vi "MC Cycle Engine Request State ERD.vi"(0 "GEA2 Reference In":refnum<k24>, 1 "GEA Inputs":T2 {"Destination" format="%.0x"; "Source" format="%.0x"}, 2 "Standalone?":bool, 7 "Cycle #":u8, 9 "MC Cycle Engine State":T1, 11 "Error In":errorcluster) -> (4 "GEA2 Reference Out":refnum<k24>, 15 "Error Out":errorcluster)   [LabVIEW 2016, in "TL27.lvlib"]
doc: "This vi can be used to update the MC cycle engine state with the requested values."
uses:
  Projects/TL27.lvlib
  C:/Automation/DLLs/PC Dot Net/GeaCommunication.dll
  Common/LabVIEW GEA2 Toolkit/LabVIEW_GEA2_Toolkit.lvlibp/type defs/Source_Destination.ctl
  type defs/MC_Cycle_Engine_Request_State.ctl
  Common/LabVIEW GEA2 Toolkit/LabVIEW_GEA2_Toolkit.lvlibp/type defs/ERD Write Data In.ctl
  Common/LabVIEW GEA2 Toolkit/LabVIEW_GEA2_Toolkit.lvlibp/type defs/Data Type.ctl
  Common/LabVIEW GEA2 Toolkit/LabVIEW_GEA2_Toolkit.lvlibp
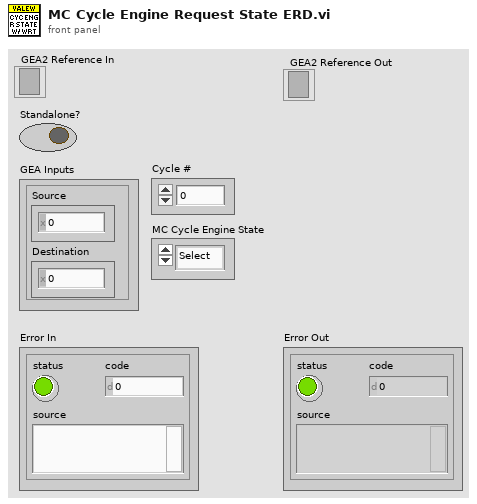
[diagram p1: front panel]
types:
  T1 = typedef "TL27.lvlib/MC_Cycle_Engine_Request_State.ctl" = enum16{"Select", "Start", "Pause", "Resume", "Stop"}
  T2 = typedef "LabVIEW_GEA2_Toolkit.lvlibp/Source_Destination.ctl" = cluster{"Source":u8, "Destination":u8}
  T3 = typedef "LabVIEW_GEA2_Toolkit.lvlibp/ERD Write Data In.ctl" = cluster{"ERD Number":u16, "Data Type":T4, "Data":string}
  T4 = typedef "LabVIEW_GEA2_Toolkit.lvlibp/Data Type.ctl" = enum16{"string", "boolean", "uint8_t", "uint16_t", "uint32_t", "uint64_t", "int8_t", "int16_t", "int32_t", "int64_t"}
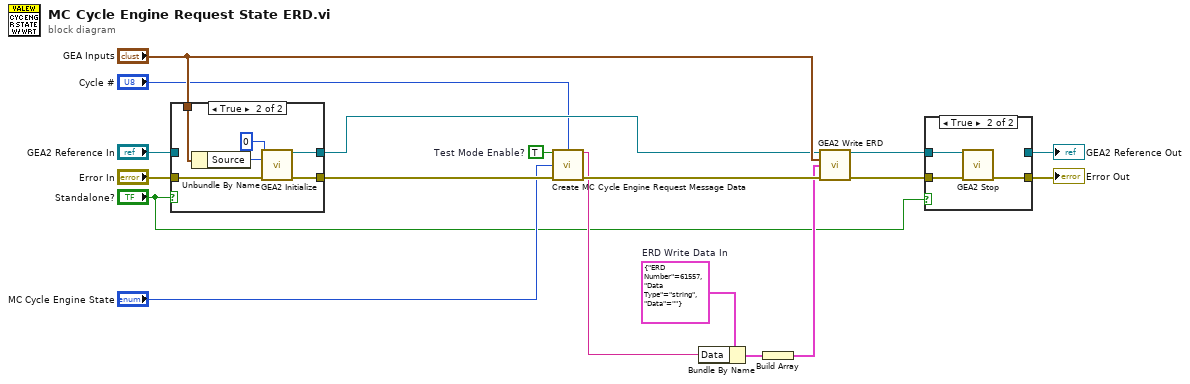
[diagram p0: block diagram]
diagram:
  w1 = TRUE  # Test Mode Enable?
  w17 = T3 {"ERD Number"=61557, "Data Type"=enum."string", "Data"=""}  # ERD Write Data In
  n1 = case shown="True" "Standalone?" {
    tunnel: "Error In" -> [w19 w26]
    tunnel: [w19 w25] -> w14
    tunnel: "GEA2 Reference In" -> [w20 _]
    tunnel: [w20 w24] -> w12
    tunnel: "GEA Inputs" -> [_ w22]
    frame False {
    }
    frame True {
      n2 = Unbundle By Name(w22) -> ("Source"=w23:u8)
      n3 = call "GEA2 Initialize.vi"("Board Index"=0, "Source Address"=w23, "error in"=w26) -> ("GEA2 Reference Out"=w24:refnum<k24>, "error out"=w25:errorcluster)  [unwired: 10 in, 1 out]
    }
  }
  n4 = call "Create MC Cycle Engine Request Message Data .vi"("Test Mode Enable?"=w1, "Cycle #"="Cycle #", "MC Cycle Engine State"="MC Cycle Engine State", "Error In"=w14) -> ("MC Cycle Engine Request Message Data"=w11:string, "Error Out"=w13:errorcluster)  [unwired: 10 in]
  n5 = Bundle By Name(cluster=w17, "Data"=w11) -> (w7:T3)
  n6 = Build Array(w7) -> (w8:T3[])
  n7 = call "GEA2 Write ERD.vi"("GEA2 Reference In"=w12, "GEA Inputs"="GEA Inputs", "Write ERD List"=w8, "Error In"=w13) -> ("GEA2 Reference Out"=w15:refnum<k24>, "Error Out"=w16:errorcluster)  [unwired: 9 in, 1 out]
  n8 = case shown="True" "Standalone?" {
    tunnel: w16 -> [w27 w31]
    tunnel: [w27 w30] -> w6
    tunnel: w15 -> [w28 w29]
    tunnel: [w28 _] -> w5
    frame False {
    }
    frame True {
      n9 = call "GEA2 Stop.vi"("GEA2 Reference In"=w29, "Error In"=w31) -> ("Error Out"=w30:errorcluster)  [unwired: 13 in]
    }
  }
  "Error Out" <- w6
  "GEA2 Reference Out" <- w5
